vi "Config Input Math.vi"(0 "VISA resource name":refnum<visa-resource-name>, 1 "Channel (1)":i32=1 min=0 max=16 step=1, 2 "Equation (0: y=mx+b)":u16(ring) items=["y=mx+b", "y=m(x+b)"], 3 "Slope(M) Value (1.000)":dbl=1.0 min=0.001 max=1000.0 step=0.001 format="%.3f", 4 "Variable B Value (0.00000E+0)":dbl min=0.0 max=100000000.0 step=1e-06 format="%^.5e", 5 "X Source (0: Kelvin)":u16(ring) items=["Kelvin", "Ohms"], 6 "B Source (0: Variable B Value)":u16(ring) items=["Variable B Value", "+Setpoint", "-Setpoint"], 7 "error in (no error)":errorcluster, 8 "Filter On/Off (F: Off)":bool, 9 "Min/Max Source (0: Kelvin)":u16(ring) items=["Kelvin", "Ohms", "Linear Data"], 10 "Settle Time (30)":dbl=30.0 min=1.0 max=200.0 step=1.0, 12 "Window (10)":dbl=10.0 min=1.0 max=80.0 step=1.0) -> (20 "VISA resource name out":refnum<visa-resource-name>, 27 "error out":errorcluster)   [LabVIEW 2012, in "Lake Shore Cryotronics 370.lvlib"]
doc: "This VI configures the math functions for the 370 inputs. Linear Equation, Min/Max, and Filter are all configured with this vi."
uses:
  <instrlib>/Lake Shore Cryotronics 370/Lake Shore Cryotronics 370.lvlib
panel:
  # "Linear Equation"
  # "Filter"
  # "Min/Max"
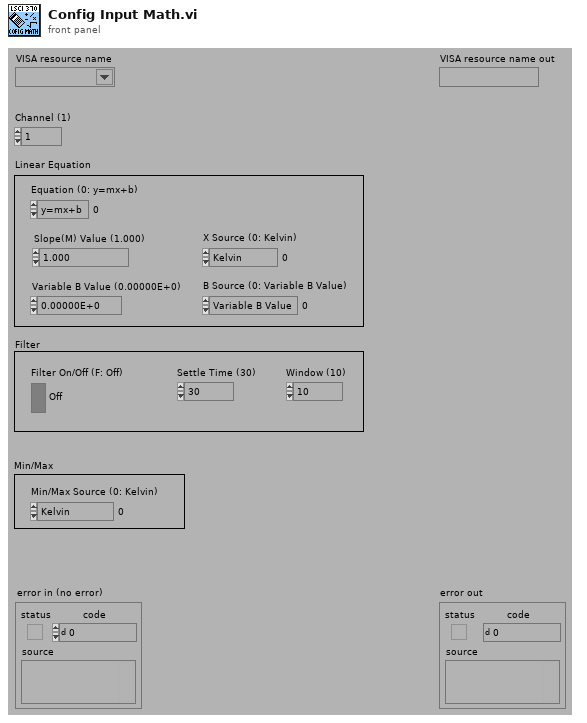
[diagram p1: front panel]
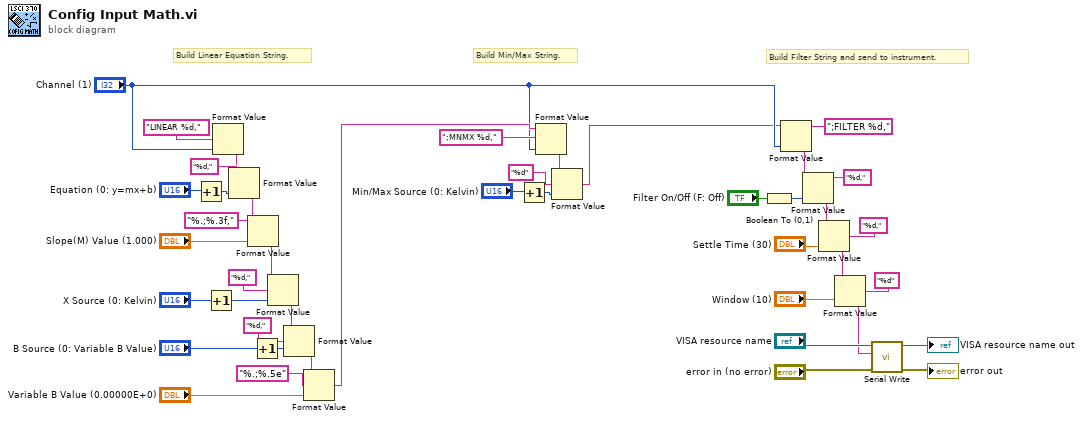
[diagram p0: block diagram]
diagram:
  # "Build Filter String and send to instrument."
  # "Build Min/Max String."
  # "Build Linear Equation String."
  n1 = Increment(x="Equation (0: y=mx+b)") -> (x+1=w31:u16)
  n2 = Increment(x="X Source (0: Kelvin)") -> (x+1=w41:u16)
  n3 = Format Value(format string="LINEAR %d,", value (0)="Channel (1)") -> (output string=w11:string)  [unwired: 1 in]
  n4 = Format Value(string ("")=w11, format string="%d,", value (0)=w31) -> (output string=w34:string)
  n5 = Format Value(string ("")=w34, format string="%.;%.3f,", value (0)="Slope(M) Value (1.000)") -> (output string=w42:string)
  n6 = Increment(x="B Source (0: Variable B Value)") -> (x+1=w36:u16)
  n7 = Format Value(string ("")=w42, format string="%d,", value (0)=w41) -> (output string=w43:string)
  n8 = Format Value(string ("")=w43, format string="%d,", value (0)=w36) -> (output string=w9:string)
  n9 = Format Value(string ("")=w9, format string="%.;%.5e", value (0)="Variable B Value (0.00000E+0)") -> (output string=w5:string)
  n10 = Increment(x="Min/Max Source (0: Kelvin)") -> (x+1=w29:u16)
  n11 = Format Value(string ("")=w5, format string=";MNMX %d,", value (0)="Channel (1)") -> (output string=w6:string)
  n12 = Format Value(string ("")=w6, format string="%d", value (0)=w29) -> (output string=w1:string)
  n13 = Boolean To (0,1)(Boolean="Filter On/Off (F: Off)") -> (0, 1=w25:i16)
  n14 = Format Value(string ("")=w1, format string=";FILTER %d,", value (0)="Channel (1)") -> (output string=w3:string)
  n15 = Format Value(string ("")=w3, format string="%d,", value (0)=w25) -> (output string=w24:string)
  n16 = Format Value(string ("")=w24, format string="%d,", value (0)="Settle Time (30)") -> (output string=w19:string)
  n17 = Format Value(string ("")=w19, format string="%d", value (0)="Window (10)") -> (output string=w14:string)
  n18 = call <instrlib>:"Serial Write.vi"("error in (no error)"="error in (no error)", "Write Buffer (\"\")"=w14, "VISA resource name"="VISA resource name") -> ("error out"=→"error out":errorcluster, "VISA resource name out"=→"VISA resource name out":refnum<visa-resource-name>)  [unwired: 6 in, 1 out]
